vi "PH_4_Pos_Selector.panel.vi"(0 "object ref":refnum<vi>, 5 "error in (no error)":errorcluster) -> (19 "error out":errorcluster)   [LabVIEW 2014, in "PH_4_Pos_Selector.lvlib"]
doc: "By this VI a ross relais can be monitored and switched. \n\nThe indicators \"CLOSED\", \"OPEN\" and \"SWITCH STATE\" show the value of the Beckhoff-Tag: blue indicates bad tag status reference problems, darkgreen false and lightgreen on. If everything is working fine, \"CLOSED\" and \"SWITCH STATE\" should show the same value, while \"OPEN\" has the opposite value. \n\nThe oval button switches the ross relais. It should be in the same state as the \"SWITCH STATE\" indicator. \n\n\"EXIT\" closes the front panel (GUI), while \"Delete Instance\" disconnects and removes the instance from the PCS.\n\nThis VI has no machine safety relevant logig: there is neither a check of internal conclict nor with other objects, for example conflict with other ross relais. Therefore it must be handled with care and should be operated by well educated operators only. It is forseen exclusively for direct operating and testing of the system. \n\nLicense Agreement for this software:\n\nCopyright (C)\nGesellschaft für Schwerionenforschung, GSI\nPlanckstr. 1\n64291 Darmstadt\nGermany\n\nContact: D.Beck@gsi.de \n\nThis program is free software; you can redistribute it and/or modify it under the terms of the GNU General Public License as published by the Free Software Foundation; either version 2 of the license, or (at your option) any later version.\n\nThis program is distributed in the hope that it will be useful, but WITHOUT ANYW ARRANTY; without even the implied warranty of MERCHANTABILITY or FITNESS FOR A PARTICULAR PURPOSE. See the GNU General License for more details (http://www.gnu.org).\n\nGesellschaft für Schwerionenforschung, GSI\nPlanckstr. 1, 64291 Darmstadt, Germany\nFor all questions and ideas contact: M.Richter@gsi.de, H.Brand@gsi.de or D.Beck@gsi.de.\nLast update: 18-DEC-2002"
uses:
  PH_4_Pos_Selector.lvlib
  PH_Basics/PH_Stepmotor_BaseClass/PH_Stepmotor_BaseClass.Axis Address.ctl
  PH_Basics/PH_Stepmotor_BaseClass/PH_Stepmotor_BaseClass.Axis Settings.ctl
  PH_Basics/PH_Stepmotor_BaseClass/PH_Stepmotor_BaseClass.Motor Type.ctl
  PH_Basics/PH_Common/Picture/PH_Picture.GUI Element 72x72.ctl
  PH_Basics/PH_Stepmotor_BaseClass/PH_Stepmotor_BaseClass.Axis Activity.ctl
  PH_Basics/PH_AxisGUI_BaseClass/PH_AxisGUI_BaseClass.Axis GUI Refs.ctl
  PH_Basics/PH_Stepmotor_BaseClass/PH_Stepmotor_BaseClass.Axis Direction.ctl
  PH_4_Pos_Selector.Position Selector.ctl
  CS_Core/CSSystem/CSSystemLib/CSSystemLib.lvlib
  PH_Basics/PH_Common/PH_Common.lvlib
  PH_Basics/PH_AxisGUI_BaseClass/PH_AxisGUI_BaseClass.lvlib
  PH_Basics/PH_Stepmotor_BaseClass/PH_Stepmotor_BaseClass.lvlib
  CS_Core/CSObj/CSObj.lvlib
  PH_AxisGUI_6P/PH_AxisGUI_6P.lvlib
  PH_Basics/PH_PSDBWriter/PH_PSDBWriter.lvlib
  PH_Basics/PH_Class/PH_Class.lvlib
panel:
  out "Activity Axis 2":T1
  out "Axis2_Status Bar":u32(colorbox) caption="Axis2"
  out "Axis2_Status":u32(colorbox)=6618880 caption="Axis2"
  out "Activity Axis 1":T1
  out "Axis1_Status Bar":u32(colorbox) caption="Axis1"
  out "Axis1_Status":u32(colorbox)=6618880 caption="Axis1"
  in  "Stop":bool caption="SetZero"
  in  "Tab Control":T2(tab)
  in  "Define Selector":i32(ring) caption="Selector"
  in  "Define Position?":bool
  in  "rel. Mode?":bool
  in  "Clear Error\nAxis 2":bool
  in  "Clear Error\nAxis 1":bool
  in  "Position IV":T3
  in  "Position III":T3
  in  "Position II":T3
  in  "Position I":T3
  in  "DOWN":bool caption="? Steps"
  in  "UP":bool caption="? Steps"
  in  "LEFT":bool caption="? Steps"
  in  "RIGHT":bool caption="? Steps"
  in  "Axis2_Target":string="0" caption="Steps"
  in  "Axis1_Target":string="0" caption="Steps"
  in  "Axis2_Settings":T4={"Sign change"=FALSE, "Width"=0.0, "Calibration"=0.0, "Unit"="Steps", "Motor Type"=enum."Unspecific", "Unit Width"="", "Unit CF"=""} caption="Axis2"
  in  "Axis1_Settings":T4={"Sign change"=FALSE, "Width"=0.0, "Calibration"=0.0, "Unit"="Steps", "Motor Type"=enum."Unspecific", "Unit Width"="", "Unit CF"=""} caption="Axis1"
  in  "AxisSelection":enum32{"Axis1", "Axis2", "Both"}(radio)=enum."Both"
  in  "SetZero":bool
  in  "Reset":bool
  out "Address Axis 1":T6={"Instance"="N/A", "Motor Nr"=0} caption="Address Axis1"
  out "Address Axis 2":T6={"Instance"="N/A", "Motor Nr"=0} caption="Address Axis2"
  out "PSDB Status":u32(colorbox)=6618880 caption="PSDB"
  in  "Delete":bool
  in  "Exit":bool
  # "PCS"
  # "3.40"
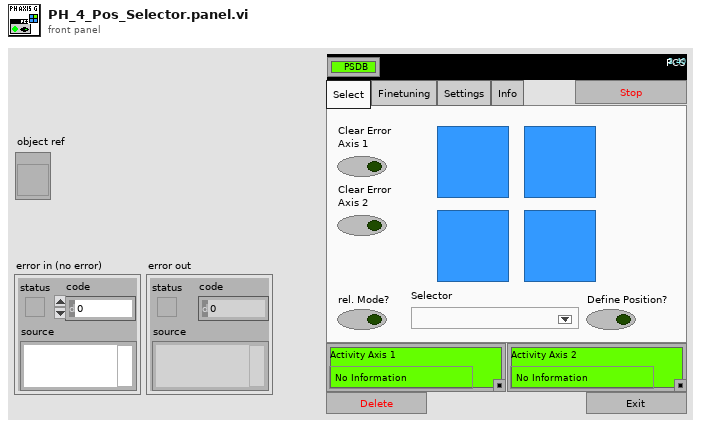
[diagram p1: front panel]
types:
  T1 = typedef "PH_Stepmotor_BaseClass.lvlib/PH_Stepmotor_BaseClass.Axis Activity.ctl" = enum16{"No Information", "stopped", "running", "Failure", "Alarm", "stopped at backward ES", "stopped at foreward ES"}
  T2 = enum32{"Select", "Finetuning", "Settings", "Info"}
  T3 = typedef "PH_Common.lvlib/PH_Picture.GUI Element 72x72.ctl" = picture
  T4 = typedef "PH_Stepmotor_BaseClass.lvlib/PH_Stepmotor_BaseClass.Axis Settings.ctl" = cluster{"Sign change":bool, "Width":dbl, "Calibration":dbl, "Unit":string, "Motor Type":T5, "Unit Width":string, "Unit CF":string}
  T5 = typedef "PH_Stepmotor_BaseClass.lvlib/PH_Stepmotor_BaseClass.Motor Type.ctl" = enum16{"Unspecific", "OWIS 49.120.2633", "OWIS 49.060.1033", "OWIS 43.040.2558", "Diamond Motion 2200 series", "OWIS 49.120.266B.MV6", "Calorimeter", "Linear Stage 1", "MICOS VT-80", "MICOS VT-80 S", "Standa Rotstage nt0.95A", "PUF RA 320.200", "PUF RA 800.200", "PUF RA 800.400", "PUF RA 400.50", "1324.nn.800.50", "1324.n9c.800.50", "1324.nn.320.200", "1324.nn.400.200", "1324.nn.800.200", "1324.nn.400.50", "1324.8c9c.800.50", "1324.8c9c.400.200"}
  T6 = typedef "PH_Stepmotor_BaseClass.lvlib/PH_Stepmotor_BaseClass.Axis Address.ctl" = cluster{"Instance":string, "Motor Nr":i32}
  T7 = typedef "PH_AxisGUI_BaseClass.lvlib/PH_AxisGUI_BaseClass.Axis GUI Refs.ctl" = cluster{"Back":refnum<vi>, "Forth":refnum<vi>, "Status":refnum<vi>, "Target":refnum<vi>, "Address":refnum<vi>, "Status Bar":refnum<vi>, "Settings":refnum<vi>, "Activity":refnum<vi>, "Clear Error":refnum<vi>}
  T8 = typedef "PH_Stepmotor_BaseClass.lvlib/PH_Stepmotor_BaseClass.Axis Direction.ctl" = enum16{"forward", "backward"}
  T9 = typedef "PH_AxisGUI_BaseClass.lvlib/PH_AxisGUI_BaseClass.i attribute.ctl" = cluster{"Axes":T10[]}
  T10 = typedef "PH_AxisGUI_BaseClass.lvlib/PH_AxisGUI_BaseClass.Axis Attributes.ctl" = cluster{"Axis GUI Refs":T7, "Address":T6, "Name":string, "Label \"Back\"":string, "Labell \"Forth\"":string, "Moving?":bool}
  T11 = typedef "PH_4_Pos_Selector.lvlib/PH_4_Pos_Selector.Position Selector.ctl" = u16
  T12 = typedef "PH_4_Pos_Selector.lvlib/PH_4_Pos_Selector.i attribute.ctl" = cluster{"GUI Refs":cluster{"Position I":refnum<vi>, "Position II":refnum<vi>, "Position III":refnum<vi>, "Position IV":refnum<vi>, "rel. Mode?":refnum<vi>, "Define Selector":refnum<vi>}, "Current Position":T11, "Service ID Position":i32, "Position Array":T13[], "Description Array":string[], "relative Mode":bool, "Wanted Define Selector Position":string}
  T13 = typedef "PH_4_Pos_Selector.lvlib/PH_4_Pos_Selector.Position.ctl" = cluster{"Axis 1":dbl, "Axis 2":dbl}
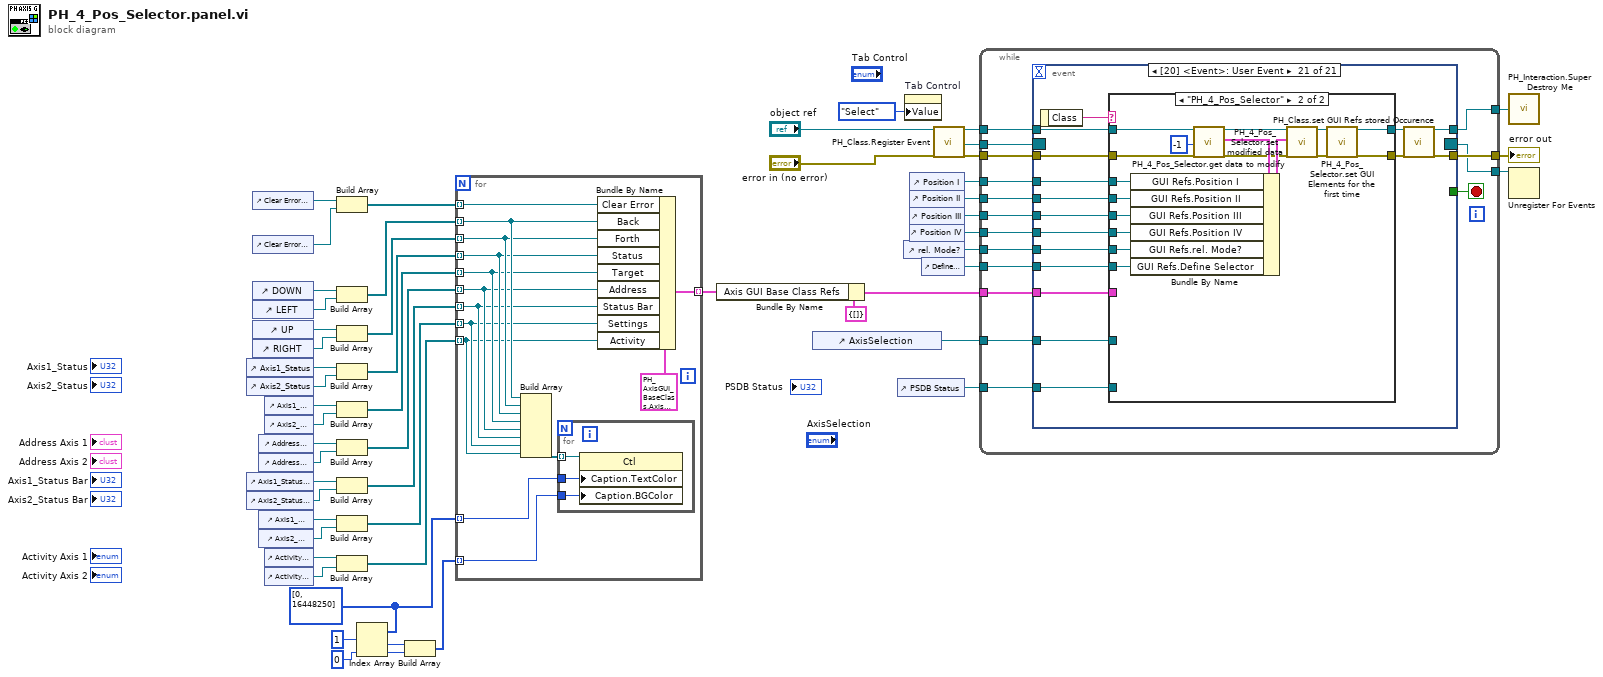
[diagram p0: block diagram]
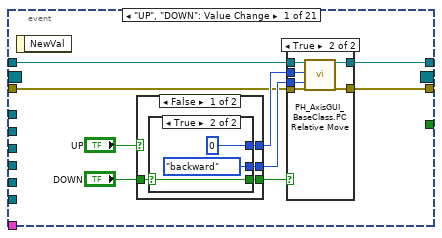
[diagram p2: hidden frame]
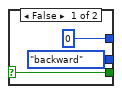
[diagram p3: hidden frame]
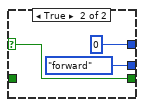
[diagram p4: hidden frame]
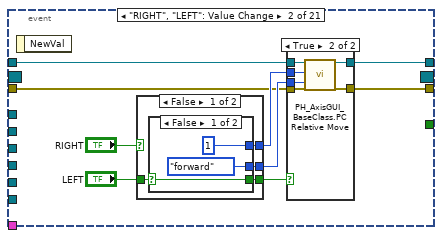
[diagram p6: hidden frame]
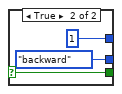
[diagram p7: hidden frame]
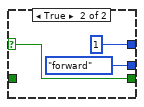
[diagram p8: hidden frame]
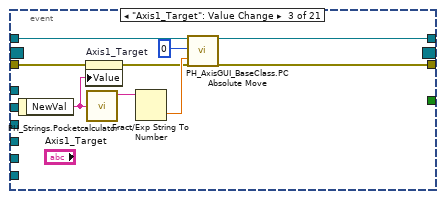
[diagram p10: hidden frame]
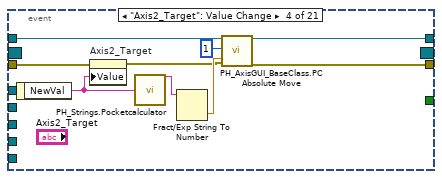
[diagram p11: hidden frame]
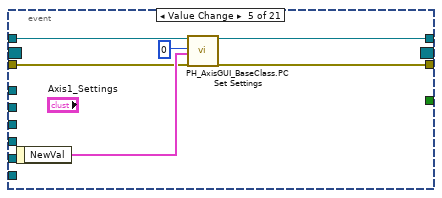
[diagram p12: hidden frame]
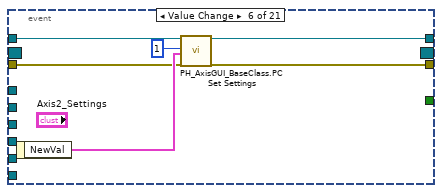
[diagram p13: hidden frame]
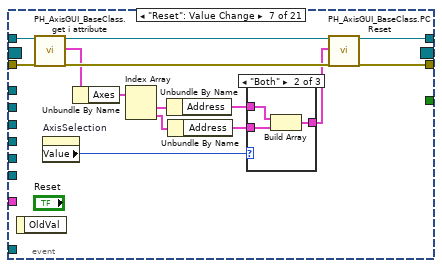
[diagram p14: hidden frame]
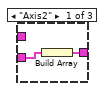
[diagram p15: hidden frame]
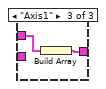
[diagram p16: hidden frame]
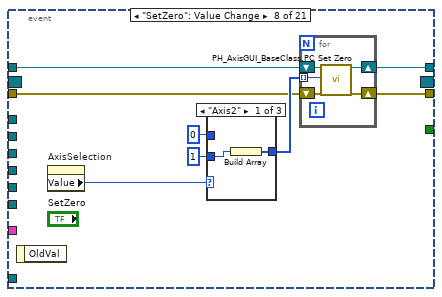
[diagram p17: hidden frame]
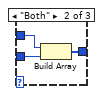
[diagram p18: hidden frame]
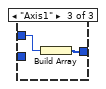
[diagram p19: hidden frame]
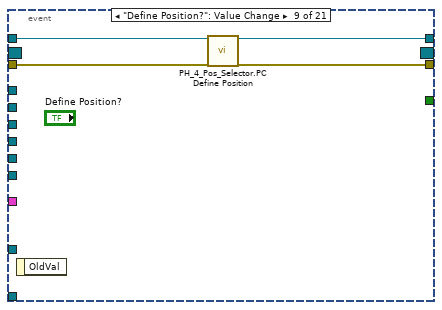
[diagram p20: hidden frame]
diagram:
  w47 = u32[] [0, 16448250]
  n1 = control-ref of="Axis1_Status"() -> (w26:refnum<vi>)
  n2 = control-ref of="Axis2_Status"() -> (w25:refnum<vi>)
  n3 = control-ref of="Axis1_Status Bar"() -> (w24:refnum<vi>)
  n4 = control-ref of="Axis2_Status Bar"() -> (w23:refnum<vi>)
  n5 = control-ref of="Clear Error\nAxis 1"() -> (w19:refnum<vi>)
  n6 = control-ref of="Clear Error\nAxis 2"() -> (w18:refnum<vi>)
  n7 = control-ref of="DOWN"() -> (w37:refnum<vi>)
  n8 = control-ref of="LEFT"() -> (w36:refnum<vi>)
  n9 = control-ref of="UP"() -> (w39:refnum<vi>)
  n10 = control-ref of="RIGHT"() -> (w38:refnum<vi>)
  n11 = control-ref of="Address Axis 1"() -> (w33:refnum<vi>)
  n12 = control-ref of="Address Axis 2"() -> (w32:refnum<vi>)
  n13 = control-ref of="Axis1_Settings"() -> (w31:refnum<vi>)
  n14 = control-ref of="Axis2_Settings"() -> (w30:refnum<vi>)
  n15 = control-ref of="Axis1_Target"() -> (w35:refnum<vi>)
  n16 = control-ref of="Axis2_Target"() -> (w34:refnum<vi>)
  n17 = control-ref of="Activity Axis 1"() -> (w22:refnum<vi>)
  n18 = control-ref of="Activity Axis 2"() -> (w21:refnum<vi>)
  n19 = Build Array(w19, w18) -> (w20:refnum<vi>[])
  n20 = Build Array(w37, w36) -> (w28:refnum<vi>[])
  n21 = Build Array(w39, w38) -> (w29:refnum<vi>[])
  n22 = Build Array(w26, w25) -> (w45:refnum<vi>[])
  n23 = Build Array(w35, w34) -> (w44:refnum<vi>[])
  n24 = Build Array(w33, w32) -> (w43:refnum<vi>[])
  n25 = Build Array(w24, w23) -> (w42:refnum<vi>[])
  n26 = Build Array(w31, w30) -> (w41:refnum<vi>[])
  n27 = Build Array(w22, w21) -> (w40:refnum<vi>[])
  n28 = Index Array(array=w47, index #1=1 ("index"), index #2=0 ("index")) -> (element #1=w49:u32, element #2=w48:u32)
  n29 = Build Array(w49, w48) -> (w46:u32[])
  n30 = for {
    tunnel: w28 -> [w65] mode=indexing
    tunnel: [w66] -> w6 mode=indexing
    tunnel: w29 -> [w64] mode=indexing
    tunnel: w45 -> [w63] mode=indexing
    tunnel: w44 -> [w62] mode=indexing
    tunnel: w43 -> [w61] mode=indexing
    tunnel: w42 -> [w60] mode=indexing
    tunnel: w41 -> [w59] mode=indexing
    tunnel: w40 -> [w55] mode=indexing
    tunnel: w46 -> [w57] mode=indexing
    tunnel: w47 -> [w56] mode=indexing
    tunnel: w20 -> [w54] mode=indexing
    n31 = Build Array(w65, w64, w63, w62, w61, w60, w59, w55) -> (w58:refnum<vi>[])
    n32 = for {
      tunnel: w58 -> [w70] mode=indexing
      tunnel: w57 -> [w69]
      tunnel: w56 -> [w68]
      n33 = property class="Ctl"(reference=w70, "Caption.TextColor"=w68, "Caption.BGColor"=w69) -> ()  [unwired: 1 in, 2 out]
    }
    n34 = Bundle By Name(cluster=T7 {"Back"=refnum, "Forth"=refnum, "Status"=refnum, "Target"=refnum, "Address"=refnum, "Status Bar"=refnum, "Settings"=refnum, "Activity"=refnum, "Clear Error"=refnum} ("GUI Refs"), "Clear Error"=w54, "Back"=w65, "Forth"=w64, "Status"=w63, "Target"=w62, "Address"=w61, "Status Bar"=w60, "Settings"=w59, "Activity"=w55) -> (w66:T7)
  }
  n35 = Bundle By Name(cluster=cluster{"Axis GUI Base Class Refs":T7[]} {"Axis GUI Base Class Refs"=[]} ("GUI Refs"), "Axis GUI Base Class Refs"=w6) -> (w3:cluster{"Axis GUI Base Class Refs":T7[]})
  n36 = control-ref of="AxisSelection"() -> (w9:refnum<vi>)
  n37 = control-ref of="PSDB Status"() -> (w8:refnum<vi>)
  n38 = control-ref of="rel. Mode?"() -> (w2:refnum<vi>)
  n39 = property on="Tab Control" class="TabCtl (strict)"("Value"=T2."Select" ("Tab Control")) -> ()  [unwired: 2 in, 2 out]
  n40 = control-ref of="Position I"() -> (w13:refnum<vi>)
  n41 = control-ref of="Position II"() -> (w12:refnum<vi>)
  n42 = control-ref of="Position III"() -> (w11:refnum<vi>)
  n43 = control-ref of="Position IV"() -> (w10:refnum<vi>)
  n44 = control-ref of="Define Selector"() -> (w1:refnum<vi>)
  n45 = call "PH_Class.Register Event.vi"("i ref in"="object ref", "error in (no error)"="error in (no error)") -> ("i ref out"=w16:refnum<vi>, "Event Registration Refnum"=w14:refnum<event-registration>, "error out"=w15:errorcluster)  [unwired: 15 in]
  n46 = while {
    tunnel: w16 -> [w83]
    tunnel: [w82] -> w53
    tunnel: w15 -> [w85]
    tunnel: [w84] -> w52
    tunnel: [w81] -> w17
    tunnel: w14 -> [w80]
    tunnel: w13 -> [w79]
    tunnel: w12 -> [w78]
    tunnel: w11 -> [w77]
    tunnel: w10 -> [w76]
    tunnel: w9 -> [w75]
    tunnel: w8 -> [w74]
    tunnel: w3 -> [w73]
    tunnel: w2 -> [w72]
    tunnel: w1 -> [w71]
    stop <- w86 stop-if-true
    n47 = event shown="[20] <Event>: User Event" {
      selector: w80 -> [_ _ _ _ _ _ _ _ _ _ _ _ _ _ _ _ _ _ _ _ _]
      dyn-events: [_ _ _ _ _ _ _ _ _ _ _ _ _ _ _ _ _ _ _ _ _] -> w81
      timeout: _ -> [_ _ _ _ _ _ _ _ _ _ _ _ _ _ _ _ _ _ _ _ _]
      tunnel: [_ _ _ _ _ _ _ _ _ _ _ _ "Delete" _ _ _ _ _ _ _ _] -> w86
      tunnel: w83 -> [w92 w122 w152 w160 w166 w173 w187 w200 w218 w224 w229 w233 w239 w242 w249 w255 w261 w267 w277 w287 w302]
      tunnel: w85 -> [w90 w120 w150 w158 w165 w172 w185 w199 w219 w223 w228 w232 w240 w241 w247 w253 w259 w265 w275 w285 w301]
      tunnel: [w89 w119 w155 w164 w170 w176 w184 w204 w220 w225 w230 w234 w236 w244 w246 w252 w258 w264 w274 w284 w292] -> w84
      tunnel: [w91 w121 w154 w163 w169 w175 w186 w205 w221 w226 w231 w235 w237 w243 w248 w254 w260 w266 w276 w286 w290] -> w82
      tunnel: w79 -> [_ _ _ _ _ _ _ _ _ _ _ _ _ _ _ _ _ _ _ _ w299]
      tunnel: w78 -> [_ _ _ _ _ _ _ _ _ _ _ _ _ _ _ _ _ _ _ _ w298]
      tunnel: w77 -> [_ _ _ _ _ _ _ _ _ _ _ _ _ _ _ _ _ _ _ _ w297]
      tunnel: w76 -> [_ _ _ _ _ _ _ _ _ _ _ _ _ _ _ _ _ _ _ _ w296]
      tunnel: w75 -> [_ _ _ _ _ _ _ _ _ _ _ _ _ _ _ _ _ _ _ _ w295]
      tunnel: w74 -> [_ _ _ _ _ _ _ _ _ _ _ _ _ _ _ _ _ _ _ _ w294]
      tunnel: w73 -> [_ _ _ _ _ _ _ _ _ _ _ _ _ _ _ _ _ _ _ _ w293]
      tunnel: w72 -> [_ _ _ _ _ _ _ _ _ _ _ _ _ _ _ _ _ _ _ _ w289]
      tunnel: w71 -> [_ _ _ _ _ _ _ _ _ _ _ _ _ _ _ _ _ _ _ _ w288]
      event "UP", "DOWN": Value Change {
        n48 = event-data() -> ()  [unwired: 1 in, 1 out]
        n49 = case shown="False" "UP" {
          selector: "UP" -> [_ w106]
          tunnel: [w99 0] -> w94
          tunnel: [w98 PH_Stepmotor_BaseClass.Axis_Direction."forward" ("direction")] -> w95
          tunnel: "DOWN" -> [w97 _]
          tunnel: [w96 w106] -> w93
          frame False {
            n50 = case shown="True" w97 {
              selector: w97 -> [w100 w103]
              tunnel: [0 0] -> w99
              tunnel: [PH_Stepmotor_BaseClass.Axis_Direction."backward" ("direction") PH_Stepmotor_BaseClass.Axis_Direction."backward" ("direction")] -> w98
              tunnel: [w100 w103] -> w96
              frame False {
              }
              frame True {
              }
            }
          }
          frame True {
          }
        }
        n51 = case shown="True" w93 {
          tunnel: w90 -> [w109 w116]
          tunnel: w92 -> [w110 w115]
          tunnel: w95 -> [_ w114]
          tunnel: [w110 w113] -> w91
          tunnel: [w109 w112] -> w89
          tunnel: w94 -> [_ w111]
          frame False {
          }
          frame True {
            n52 = call "PH_AxisGUI_BaseClass.PC Relative Move.vi"("i ref in"=w115, "Axis"=w111, "direction"=w114, "error in"=w116) -> ("i ref out"=w113:refnum<vi>, "error out"=w112:errorcluster)  [unwired: 14 in]
          }
        }
      }
      event "RIGHT", "LEFT": Value Change {
        n53 = event-data() -> ()  [unwired: 1 in, 1 out]
        n54 = case shown="False" "RIGHT" {
          selector: "RIGHT" -> [_ w136]
          tunnel: [w129 1] -> w124
          tunnel: [w128 PH_Stepmotor_BaseClass.Axis_Direction."forward" ("direction")] -> w125
          tunnel: "LEFT" -> [w127 _]
          tunnel: [w126 w136] -> w123
          frame False {
            n55 = case shown="False" w127 {
              selector: w127 -> [w130 w133]
              tunnel: [1 1] -> w129
              tunnel: [PH_Stepmotor_BaseClass.Axis_Direction."forward" ("direction") PH_Stepmotor_BaseClass.Axis_Direction."backward" ("direction")] -> w128
              tunnel: [w130 w133] -> w126
              frame False {
              }
              frame True {
              }
            }
          }
          frame True {
          }
        }
        n56 = case shown="True" w123 {
          tunnel: w120 -> [w139 w146]
          tunnel: w122 -> [w140 w145]
          tunnel: w125 -> [_ w144]
          tunnel: [w140 w143] -> w121
          tunnel: [w139 w142] -> w119
          tunnel: w124 -> [_ w141]
          frame False {
          }
          frame True {
            n57 = call "PH_AxisGUI_BaseClass.PC Relative Move.vi"("i ref in"=w145, "Axis"=w141, "direction"=w144, "error in"=w146) -> ("i ref out"=w143:refnum<vi>, "error out"=w142:errorcluster)  [unwired: 14 in]
          }
        }
      }
      event "Axis1_Target": Value Change {
        n58 = event-data() -> ("NewVal"=w147:string)  [unwired: 1 in]
        n59 = property on="Axis1_Target" class="Str"(error in=w150, "Value"=w147) -> (error out=w148:errorcluster)  [unwired: 1 in, 1 out]
        n60 = call "PH_Strings.Pocketcalculator.vi"("Input"=w147) -> ("String Double"=w153:string)  [unwired: 3 out]
        n61 = Fract/Exp String To Number(string=w153) -> (number=w149:dbl)  [unwired: 3 in, 1 out]
        n62 = call "PH_AxisGUI_BaseClass.PC Absolute Move.vi"("i ref in"=w152, "Axis"=0, "Position [Units]"=w149, "error in"=w148) -> ("i ref out"=w154:refnum<vi>, "error out"=w155:errorcluster)  [unwired: 14 in]
      }
      event "Axis2_Target": Value Change {
        n63 = event-data() -> ("NewVal"=w156:string)  [unwired: 1 in]
        n64 = property on="Axis2_Target" class="Str"(error in=w158, "Value"=w156) -> (error out=w157:errorcluster)  [unwired: 1 in, 1 out]
        n65 = call "PH_Strings.Pocketcalculator.vi"("Input"=w156) -> ("String Double"=w162:string)  [unwired: 3 out]
        n66 = Fract/Exp String To Number(string=w162) -> (number=w161:dbl)  [unwired: 3 in, 1 out]
        n67 = call "PH_AxisGUI_BaseClass.PC Absolute Move.vi"("i ref in"=w160, "Axis"=1, "Position [Units]"=w161, "error in"=w157) -> ("i ref out"=w163:refnum<vi>, "error out"=w164:errorcluster)  [unwired: 14 in]
      }
      event Value Change {
        n68 = event-data() -> ("NewVal"=w168:T4)  [unwired: 1 in]
        n69 = call "PH_AxisGUI_BaseClass.PC Set Settings.vi"("VI in"=w166, "Axis"=0, "NewVal"=w168, "error in (no error)"=w165) -> ("VI out"=w169:refnum<vi>, "error out"=w170:errorcluster)  [unwired: 14 in]
      }
      event Value Change {
        n70 = event-data() -> ("NewVal"=w174:T4)  [unwired: 1 in]
        n71 = call "PH_AxisGUI_BaseClass.PC Set Settings.vi"("VI in"=w173, "Axis"=1, "NewVal"=w174, "error in (no error)"=w172) -> ("VI out"=w175:refnum<vi>, "error out"=w176:errorcluster)  [unwired: 14 in]
      }
      event "Reset": Value Change {
        n72 = event-data() -> ()  [unwired: 1 in, 1 out]
        n73 = call "PH_AxisGUI_BaseClass.get i attribute.vi"("i ref in"=w187, "error in (no error)"=w185) -> ("i ref out"=w189:refnum<vi>, "i attribute"=w183:T9, "error out"=w190:errorcluster)  [unwired: 15 in]
        n74 = property on="AxisSelection" class="RadioBtnsControl (strict)"() -> ("Value"=w177:enum32{"Axis1", "Axis2", "Both"})  [unwired: 2 in, 2 out]
        n75 = Unbundle By Name(w183) -> ("Axes"=w182:T10[])
        n76 = Index Array(array=w182) -> (element #1=w181:T10, element #2=w180:T10)  [unwired: 2 in]
        n77 = Unbundle By Name(w181) -> ("Address"=w178:T6)
        n78 = Unbundle By Name(w180) -> ("Address"=w179:T6)
        n79 = case shown="\"Both\"" w177 {
          tunnel: [w192 w195 w197] -> w188
          tunnel: w179 -> [w191 w194 _]
          tunnel: w178 -> [_ w193 w196]
          frame "Axis2" {
            n80 = Build Array(w191) -> (w192:T6[])
          }
          frame "Both" {
            n81 = Build Array(w193, w194) -> (w195:T6[])
          }
          frame "Axis1" {
            n82 = Build Array(w196) -> (w197:T6[])
          }
        }
        n83 = call "PH_AxisGUI_BaseClass.PC Reset.vi"("i ref in"=w189, "Addresses"=w188, "error in"=w190) -> ("i ref out"=w186:refnum<vi>, "error out"=w184:errorcluster)  [unwired: 15 in]
      }
      event "SetZero": Value Change {
        n84 = event-data() -> ()  [unwired: 1 in, 1 out]
        n85 = property on="AxisSelection" class="RadioBtnsControl (strict)"() -> ("Value"=w198:enum32{"Axis1", "Axis2", "Both"})  [unwired: 2 in, 2 out]
        n86 = case shown="\"Axis2\"" w198 {
          tunnel: [w212 w215 w217] -> w203
          tunnel: 1 -> [w211 w214 _]
          tunnel: 0 -> [_ w213 w216]
          frame "Axis2" {
            n87 = Build Array(w211) -> (w212:i32[])
          }
          frame "Both" {
            n88 = Build Array(w213, w214) -> (w215:i32[])
          }
          frame "Axis1" {
            n89 = Build Array(w216) -> (w217:i32[])
          }
        }
        n90 = for {
          tunnel: w203 -> [w206] mode=indexing
          shift-right: [w207] -> w204
          shift-left: w199 -> [w210]
          shift-right: [w208] -> w205
          shift-left: w200 -> [w209]
          n91 = call "PH_AxisGUI_BaseClass.PC Set Zero.vi"("VI in"=w209, "Axis"=w206, "error in (no error)"=w210) -> ("VI out"=w208:refnum<vi>, "error out"=w207:errorcluster)  [unwired: 15 in]
        }
      }
      event "Define Position?": Value Change {
        n92 = event-data() -> ()  [unwired: 1 in, 1 out]
        n93 = call "PH_4_Pos_Selector.PC Define Position.vi"("VI in"=w218, "error in (no error)"=w219) -> ("VI out"=w221:refnum<vi>, "error out"=w220:errorcluster)  [unwired: 16 in]
      }
      event "Clear Error\nAxis 1": Value Change {
        n94 = event-data() -> ()  [unwired: 1 in, 1 out]
        n95 = call "PH_AxisGUI_BaseClass.PC Clear Error.vi"("i ref in"=w224, "Axis"=0, "error in"=w223) -> ("i ref out"=w226:refnum<vi>, "error out"=w225:errorcluster)  [unwired: 15 in]
      }
      event "Clear Error\nAxis 2": Value Change {
        n96 = event-data() -> ()  [unwired: 1 in, 1 out]
        n97 = call "PH_AxisGUI_BaseClass.PC Clear Error.vi"("i ref in"=w229, "Axis"=1, "error in"=w228) -> ("i ref out"=w231:refnum<vi>, "error out"=w230:errorcluster)  [unwired: 15 in]
      }
      event "Stop": Value Change {
        n98 = event-data() -> ()  [unwired: 1 in, 1 out]
        n99 = call "PH_AxisGUI_BaseClass.PC Stop.vi"("VI in"=w233, "error in (no error)"=w232) -> ("VI out"=w235:refnum<vi>, "error out"=w234:errorcluster)  [unwired: 16 in]
      }
      event "Delete": Value Change {
        n100 = event-data() -> ()  [unwired: 1 in, 1 out]
        n101 = call "PH_Class.Delete GUI.vi"("VI in"=w239, "error in (no error)"=w240) -> ("VI out"=w237:refnum<vi>, "error out"=w236:errorcluster)  [unwired: 16 in]
      }
      event "Exit": Value Change {
        n102 = event-data() -> ()  [unwired: 1 in, 1 out]
        n103 = call "CSObj.open front panel.vi"("i ref in"=w242, "frontPanelOpen"=FALSE ("front panel open"), "error in (no error)"=w241) -> ("i ref out"=w243:refnum<vi>, "error out"=w244:errorcluster)  [unwired: 15 in]
      }
      event Mouse Up {
        w250 = T11 1 items=["unknown", "Position I", "Position II", "Position III", "Position IV"] ("Wanted Position")
        n104 = event-data() -> ()  [unwired: 1 in, 1 out]
        n105 = call "CSSystemLib.ref2name.vi"("obj refnum"=w249) -> ("name"=w251:string)
        n106 = call "PH_4_Pos_Selector.Evt Call Select Position.vi"("i ref in"=w249, "4 Pos instance"=w251, "Wanted Position"=w250, "error in"=w247) -> ("i ref out"=w248:refnum<vi>, "error out"=w246:errorcluster)  [unwired: 14 in]
      }
      event Mouse Up {
        w256 = T11 2 items=["unknown", "Position I", "Position II", "Position III", "Position IV"] ("Wanted Position")
        n107 = event-data() -> ()  [unwired: 1 in, 1 out]
        n108 = call "CSSystemLib.ref2name.vi"("obj refnum"=w255) -> ("name"=w257:string)
        n109 = call "PH_4_Pos_Selector.Evt Call Select Position.vi"("i ref in"=w255, "4 Pos instance"=w257, "Wanted Position"=w256, "error in"=w253) -> ("i ref out"=w254:refnum<vi>, "error out"=w252:errorcluster)  [unwired: 14 in]
      }
      event Mouse Up {
        w262 = T11 3 items=["unknown", "Position I", "Position II", "Position III", "Position IV"] ("Wanted Position")
        n110 = event-data() -> ()  [unwired: 1 in, 1 out]
        n111 = call "CSSystemLib.ref2name.vi"("obj refnum"=w261) -> ("name"=w263:string)
        n112 = call "PH_4_Pos_Selector.Evt Call Select Position.vi"("i ref in"=w261, "4 Pos instance"=w263, "Wanted Position"=w262, "error in"=w259) -> ("i ref out"=w260:refnum<vi>, "error out"=w258:errorcluster)  [unwired: 14 in]
      }
      event Mouse Up {
        w268 = T11 4 items=["unknown", "Position I", "Position II", "Position III", "Position IV"] ("Wanted Position")
        n113 = event-data() -> ()  [unwired: 1 in, 1 out]
        n114 = call "CSSystemLib.ref2name.vi"("obj refnum"=w267) -> ("name"=w269:string)
        n115 = call "PH_4_Pos_Selector.Evt Call Select Position.vi"("i ref in"=w267, "4 Pos instance"=w269, "Wanted Position"=w268, "error in"=w265) -> ("i ref out"=w266:refnum<vi>, "error out"=w264:errorcluster)  [unwired: 14 in]
      }
      event "rel. Mode?": Value Change {
        n116 = event-data() -> ("CtlRef"=w271:refnum<vi>, "OldVal"=w270:bool, "NewVal"=w273:bool)  [unwired: 1 in]
        n117 = property class="Bool (strict)"(reference=w271, error in=w275, "Value"=w270) -> (error out=w272:errorcluster)  [unwired: 1 out]
        n118 = call "CSSystemLib.ref2name.vi"("obj refnum"=w277) -> ("name"=w278:string)
        n119 = call "PH_4_Pos_Selector.Evt Call Relative Mode.vi"("i ref in"=w277, "4 Pos instance"=w278, "Relative Mode?"=w273, "error in"=w272) -> ("i ref out"=w276:refnum<vi>, "error out"=w274:errorcluster)  [unwired: 14 in]
      }
      event "Define Selector": Value Change {
        n120 = event-data() -> ("CtlRef"=w282:refnum<vi>)  [unwired: 1 in]
        n121 = property class="Ring (strict)"(reference=w282, error in=w285) -> (error out=w283:errorcluster, "Strings []"=w281:string[], "Value"=w280:i32)  [unwired: 1 out]
        n122 = Index Array(array=w281, index=w280) -> (element=w279:string)
        n123 = call "PH_4_Pos_Selector.PC set wanted define selector position.vi"("VI in"=w287, "Wanted Define Selector Position"=w279, "error in (no error)"=w283) -> ("VI out"=w286:refnum<vi>, "error out"=w284:errorcluster)  [unwired: 15 in]
      }
      event User Event {
        n124 = event-data() -> ("Class"=w303:string)  [unwired: 1 in]
        n125 = case shown="\"PH_4_Pos_Selector\"" w303 {
          selector: w303 -> [w305 _]
          tunnel: w302 -> [w313 w325]
          tunnel: [w308 w315] -> w291
          tunnel: w301 -> [w312 w324]
          tunnel: [w306 w317] -> w300
          tunnel: w299 -> [_ w323]
          tunnel: w298 -> [_ w322]
          tunnel: w297 -> [_ w321]
          tunnel: w296 -> [_ w320]
          tunnel: w295 -> [w311 _]
          tunnel: w294 -> [w304 _]
          tunnel: w293 -> [w310 _]
          tunnel: w289 -> [_ w318]
          tunnel: w288 -> [_ w314]
          frame Default {
            n126 = call "PH_AxisGUI_6P.set GUI Refs.vi"("i ref in"=w313, "Class"=w305, "GUI Refs"=w310, "AxisSelection"=w311, "error in"=w312) -> ("i ref out"=w309:refnum<vi>, "error out"=w307:errorcluster)  [unwired: 13 in]
            n127 = call "PH_PSDBWriter.set GUI Refs.vi"("i ref in"=w309, "Class"=w305, "Ref PSDB Status"=w304, "error in"=w307) -> ("i ref out"=w308:refnum<vi>, "error out"=w306:errorcluster)  [unwired: 14 in]
          }
          frame "PH_4_Pos_Selector" {
            n128 = call "PH_4_Pos_Selector.get data to modify.vi"("i ref in"=w325, "ms timeout (10000)"=-1, "error in (no error)"=w324) -> ("i ref out"=w327:refnum<vi>, "i attribute"=w328:T12, "error out"=w326:errorcluster)  [unwired: 13 in, 1 out]
            n129 = Bundle By Name(cluster=w328, "GUI Refs.Position I"=w323, "GUI Refs.Position II"=w322, "GUI Refs.Position III"=w321, "GUI Refs.Position IV"=w320, "GUI Refs.rel. Mode?"=w318, "GUI Refs.Define Selector"=w314) -> (w330:T12)
            n130 = call "PH_4_Pos_Selector.set modified data.vi"("i ref in"=w327, "i attribute"=w330, "error in (no error)"=w326) -> ("i ref out"=w316:refnum<vi>, "error out"=w319:errorcluster)  [unwired: 15 in]
            n131 = call "PH_4_Pos_Selector.set GUI Elements for the first time.vi"("VI in"=w316, "error in (no error)"=w319) -> ("VI out"=w315:refnum<vi>, "error out"=w317:errorcluster)  [unwired: 16 in]
          }
        }
        n132 = call "PH_Class.set GUI Refs stored Occurence.vi"("i ref in"=w291, "error in (no error)"=w300) -> ("i ref out"=w290:refnum<vi>, "error out"=w292:errorcluster)  [unwired: 16 in]
      }
    }
  }
  "error out" <- w52
  n133 = call "PH_Interaction.Super Destroy Me.vi"("i ref out"=w53) -> ()
  n134 = Unregister For Events(event registration refnum=w17) -> ()  [unwired: 1 in, 1 out]
